vi "Hub Read.vi"(4 "timeout ms (25000)":i32=250000, 6 "Bytes per sample":i32=4, 8 "error in (no error)":errorcluster, 9 "hub port":u64=2, 10 "Number of samples":u64, 11 "RP Communicator in":refnum<class "RP Communicator.lvclass">) -> (0 "error out":errorcluster, 2 "data out":string, 3 "RP Communicator out":refnum<class "RP Communicator.lvclass">)   [LabVIEW 2024, in "RP Communicator.lvclass"]
uses:
  RP Communicator.lvclass
  RP Communicator.lvclass/RP Communicator.ctl
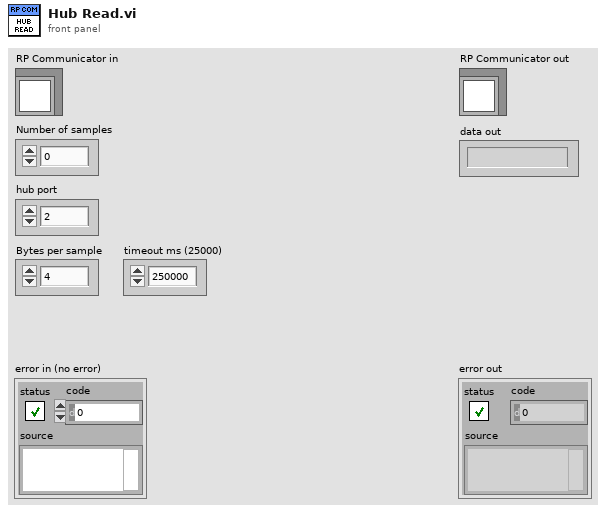
[diagram p1: front panel]
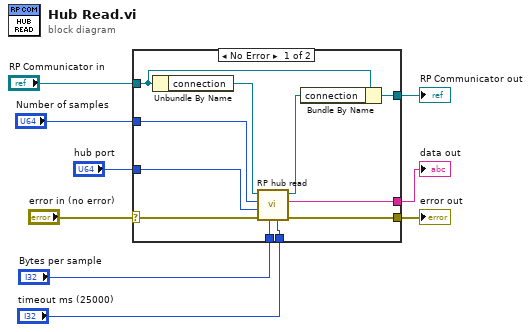
[diagram p0: block diagram]
diagram:
  n1 = case shown="No Error" "error in (no error)" {
    selector: "error in (no error)" -> [w15 w22]
    tunnel: [w16 w22] -> w8
    tunnel: [w18 w21] -> w6
    tunnel: "RP Communicator in" -> [w20 w21]
    tunnel: "Number of samples" -> [w14 _]
    tunnel: "hub port" -> [w13 _]
    tunnel: [w12 _] -> w3
    tunnel: "Bytes per sample" -> [w11 _]
    tunnel: "timeout ms (25000)" -> [w10 _]
    frame No Error {
      n2 = Unbundle By Name(w20) -> ("connection"=w19:refnum<k5>)
      n3 = call "RP hub read.vi"("timeout ms (25000)"=w10, "Bytes per sample"=w11, "Error In"=w15, "hub port"=w13, "Number of samples"=w14, "connection ID"=w19) -> ("Error Out"=w16:errorcluster, "data out"=w12:string, "connection ID out"=w17:refnum<k5>)  [unwired: 3 in]
      n4 = Bundle By Name(cluster=w20, "connection"=w17) -> (w18:refnum<class "RP Communicator.lvclass">)
    }
    frame Error {
    }
  }
  "error out" <- w8
  "RP Communicator out" <- w6
  "data out" <- w3
